vi "RSDC-триггер.vi"(2 "S":bool, 3 "C":bool, 4 "D":bool, 5 "R":bool) -> (0 "not Q":bool, 1 "Q":bool)   [LabVIEW 2012]
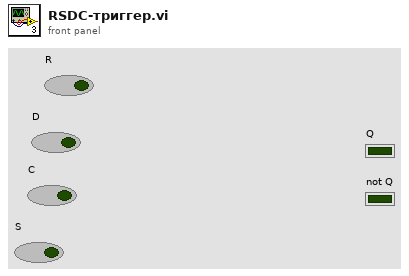
[diagram p1: front panel]
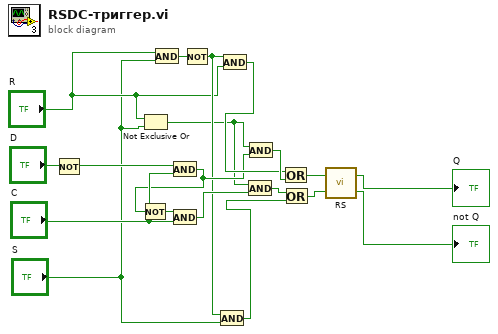
[diagram p0: block diagram]
diagram:
  n1 = Not(x="D") -> (.not. x?=w16:bool)
  n2 = Not Exclusive Or(1:"S", 2:"R") -> (0:w5:bool)
  n3 = And(x="R", y="S") -> (x .and. y?=w15:bool)
  n4 = And(x=w16, y="C") -> (x .and. y?=w10:bool)
  n5 = Not(x=w10) -> (.not. x?=w18:bool)
  n6 = And(x=w18, y="C") -> (x .and. y?=w9:bool)
  n7 = Not(x=w15) -> (.not. x?=w8:bool)
  n8 = And(x=w8, y="S") -> (x .and. y?=w14:bool)
  n9 = And(x=w8, y="R") -> (x .and. y?=w11:bool)
  n10 = And(x=w5, y=w9) -> (x .and. y?=w13:bool)
  n11 = And(x=w5, y=w10) -> (x .and. y?=w12:bool)
  n12 = Or(x=w11, y=w12) -> (x .or. y?=w4:bool)
  n13 = Or(x=w13, y=w14) -> (x .or. y?=w3:bool)
  n14 = call "RS.vi"("S"=w3, "R"=w4) -> ("not Q"=→"not Q":bool, "Q"=→"Q":bool)
